vi "Is Valid File.vi"(8 "Error In":errorcluster, 11 "File":path) -> (0 "Error Out":errorcluster, 2 "Valid file":bool, 3 "File out":path)   [LabVIEW 2019]
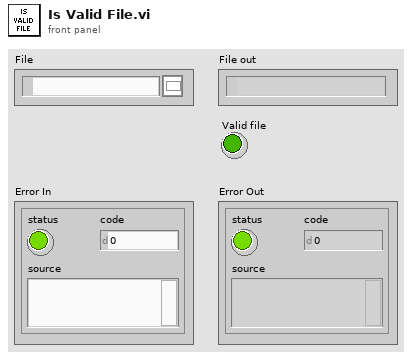
[diagram p1: front panel]
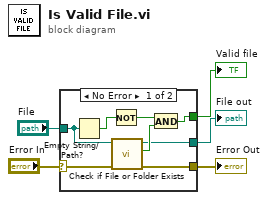
[diagram p0: block diagram]
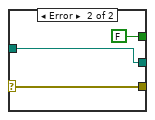
[diagram p2: hidden frame]
diagram:
  n1 = case shown="No Error" "Error In" {
    selector: "Error In" -> [w6 w16]
    tunnel: [w10 w16] -> w5
    tunnel: [w9 w15] -> w4
    tunnel: "File" -> [w8 w15]
    tunnel: [w7 FALSE] -> w2
    frame No Error {
      n2 = Empty String/Path?(string/path=w8) -> (empty?=w11:bool)
      n3 = Not(x=w11) -> (.not. x?=w12:bool)
      n4 = call <vilib>:"Check if File or Folder Exists.vi"("error in (no error)"=w6, "path"=w8) -> ("error out"=w10:errorcluster, "file or folder exists?"=w13:bool, "dup path"=w9:path)  [unwired: 7 in]
      n5 = And(x=w12, y=w13) -> (x .and. y?=w7:bool)
    }
    frame Error {
    }
  }
  "Error Out" <- w5
  "File out" <- w4
  "Valid file" <- w2
